vi "SP Simulate Filter Data.vi"() -> ()   [LabVIEW 2011]
uses:
  TypeDefs/SP Filter Type.ctl
panel:
  in  "Points":i32=181
  in  "Filter Type":T1=enum."Bandpass"
  out "X Values":i32[](array[numeric])=[0, 1, 2, 3, 4, 5, 6, 7, 8, 9, 10, 11, 12, 13, 14, 15, 16, 17, 18, 19, 20, 21, 22, 23, 24, 25, 26, 27, 28, 29, 30, 31, 32, 33, 34, 35, 36, 37, 38, 39, 40, 41, 42, 43, 44, 45, 46, 47, 48, 49, 50, 51, 52, 53, 54, 55, 56, 57, 58, 59, 60, 61, 62, 63, 64, 65, 66, 67, 68, 69, 70, 71, 72, 73, 74, 75, 76, 77, 78, 79, 80, 81, 82, 83, 84, 85, 86, 87, 88, 89, 90, 91, 92, 93, 94, 95, 96, 97, 98, 99, 100, 101, 102, 103, 104, 105, 106, 107, 108, 109, 110, 111, 112, 113, 114, 115, 116, 117, 118, 119, 120, 121, 122, 123, 124, 125, 126, 127, 128, 129, 130, 131, 132, 133, 134, 135, 136, 137, 138, 139, 140, 141, 142, 143, 144, 145, 146, 147, 148, 149, 150, 151, 152, 153, 154, 155, 156, 157, 158, 159, 160, 161, 162, 163, 164, 165, 166, 167, 168, 169, 170, 171, 172, 173, 174, 175, 176, 177, 178, 179, 180, 181, 182, 183, 184, 185, 186, 187, 188, 189, 190, 191, 192, 193, 194, 195, 196, 197, 198, 199, 200]
  out "Y Values":dbl[](array[numeric])=[-6.0, -6.0, -6.0, -6.0, -6.0, -6.0, -5.0, -4.0, -3.0, -2.0, -1.1855130217753456, -0.9392889870179464, -1.1861908270355541, -1.1367726789453658, -1.0393042985006378, -1.1729735369456953, -1.149385365911845, -1.1147598905277212, -0.8924252750804288, -0.852023103699543, -1.0009058190824704, -1.1663956046137898, -0.9001054770728154, -1.130526922084043, -1.1865443801186122, -0.8041911034172179, -1.1354203858940595, -0.9810522632655637, -0.8174498820167059, -0.8314370257909104, -1.1470623100787634, -0.8322674500080469, -1.139672707857633, -1.1197357445850977, -0.9958965192526265, -0.9621243610180682, -1.0476905954524998, -0.8242021422725134, -1.1913494829905178, -0.9868466615040767, -1.1724387156436977, -1.167152572929662, -0.8616430603149867, -1.140654519892024, -0.8539829798042038, -0.9647720176391821, -0.8587315795201268, -1.0567091604204648, -1.1192572463176262, -0.98486077165281, -1.0198831233507435, -1.0453093341117357, -0.9090367415909884, -0.9225201376325742, -0.8147168036204276, -1.107631457719548, -0.8164589952129693, -1.0035047526744438, -0.9758160980658377, -1.184168855175436, -0.842430499284283, -0.8295055444174504, -1.0907174559726884, -1.0463289127086592, -0.9523684118905202, -1.0086763511633476, -1.0058400904040357, -1.0432787022227192, -1.0004346015349277, -1.0142579998073553, -1.03249973907765, -1.1571657456698485, -0.8532729270453172, -0.830847736139528, -0.8321614396956182, -0.8398525997752223, -1.0931777911207057, -0.9353850412309945, -1.1033135631481505, -0.8359862020321329, -1.0100917820568274, -0.9437528106627642, -0.9234950263145335, -1.1828469590895319, -0.9732178966488259, -0.8312094485882828, -1.0994433199614881, -1.0711340736405945, -1.0161854731131412, -1.057480045668262, -1.0787569146834337, -1.150715751536042, -0.9306538142740585, -0.8619442330284444, -0.9498060661557108, -0.8760250798284357, -0.9560421828466075, -0.9006082904852345, -0.9198347197329708, -1.0706736281223097, -0.9910446023988131, -1.1659285288433643, -1.0742803411609738, -0.9771859793673917, -0.9576780670324955, -0.8573848364754029, -0.987301020537021, -0.815083398408206, -0.9954303077443712, -0.904598633827661, -0.917020167248773, -0.9859233342771836, -1.0886427454423657, -0.824049503823506, -0.9267990550448937, -1.0502624782226144, -0.9990423620181306, -0.9308037411565736, -1.1098504590826779, -1.159288905649198, -1.151169461672428, -0.8979842313793596, -1.0781960839410027, -1.0969866075108148, -1.113520232849719, -0.9242437596372882, -0.8322010245145881, -0.9131005811595208, -1.0502624924705835, -0.9860920827871864, -0.9686948150309891, -1.0436064687859832, -0.9811735822378999, -0.918340390858149, -1.087828104328058, -0.9581834504413268, -0.9790485893409894, -0.91805118027203, -0.8394459605871857, -1.0587904780939332, -1.1043679940556488, -1.103235946130976, -0.9329546049267435, -1.0870438319895284, -0.869725151175479, -0.8527906822295972, -0.8936094898921996, -0.8623252114256822, -1.0839364126457178, -1.1610235966131799, -1.0852518226294485, -0.8429280021959311, -1.1856901887322082, -1.052078336001964, -1.1295501456348471, -1.014702536100275, -1.107668899453921, -0.808453691868899, -1.0741488503523051, -1.0676276895458034, -0.8050463016216658, -0.9702859338685449, -1.037849817531343, -1.1042259704060462, -1.087009412780065, -0.9269022138105869, -0.8821968384650177, -0.9952550757996109, -1.0399315437270453, -1.1993212651287672, -1.1661312738652736, -1.0812208427752024, -1.1971807752359445, -1.1135450915006633, -0.8193764144655277, -0.9009947308628669, -0.8717741642808872, -1.007749740491375, -0.896481392578258, -0.964590014671117, -1.106404269705894, -1.0422703718848416, -0.9463098078312262, -1.0200691923673444, -1.056772196366392, -0.9059923317295363, -0.9680609411906224, -0.8086586664793829, -0.8983537306170685, -1.1283136612464237, -1.117694602097225, -2.0, -3.0, -4.0, -5.0, -6.0, -6.0, -6.0, -6.0, -6.0, -6.0]
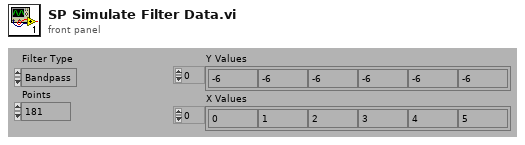
[diagram p1: front panel]
types:
  T1 = typedef "SP Filter Type.ctl" = enum16{"Lowpass", "Highpass", "Bandpass", "Bandstop"}
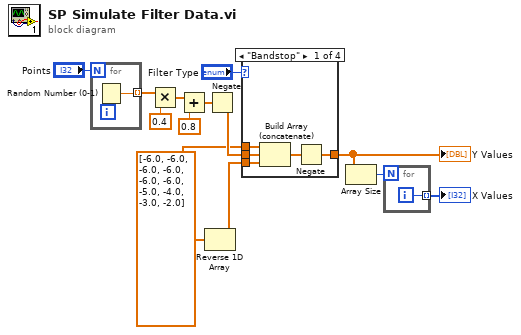
[diagram p0: block diagram]
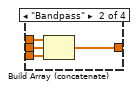
[diagram p2: hidden frame]
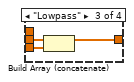
[diagram p3: hidden frame]
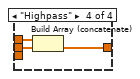
[diagram p4: hidden frame]
diagram:
  w4 = dbl[] [-6.0, -6.0, -6.0, -6.0, -6.0, -6.0, -5.0, -4.0, -3.0, -2.0] ("x+y")
  n1 = for {
    N: "Points" -> [_]
    tunnel: [w14] -> w12 mode=indexing
    n2 = Random Number (0-1)() -> (number: 0 to 1=w14:dbl)
  }
  n3 = Multiply(x=w12, y=0.4 ("number: 0 to 1")) -> (x*y=w10:dbl[])
  n4 = Add(x=w10, y=0.8 ("number: 0 to 1")) -> (x+y=w8:dbl[])
  n5 = Reverse 1D Array(array=w4) -> (reversed array=w3:dbl[])
  n6 = Negate(x=w8) -> (-x=w7:dbl[])
  n7 = case shown="\"Bandstop\"" "Filter Type" {
    tunnel: w7 -> [w19 w23 w26 w29]
    tunnel: w4 -> [w18 w22 _ w27]
    tunnel: w3 -> [w17 w21 w25 _]
    tunnel: [w15 w20 w24 w28] -> w2
    frame "Bandstop" {
      n8 = Build Array (concatenate)(w18, w19, w17) -> (w16:dbl[])
      n9 = Negate(x=w16) -> (-x=w15:dbl[])
    }
    frame "Bandpass" {
      n10 = Build Array (concatenate)(w22, w23, w21) -> (w20:dbl[])
    }
    frame "Lowpass" {
      n11 = Build Array (concatenate)(w26, w25) -> (w24:dbl[])
    }
    frame "Highpass" {
      n12 = Build Array (concatenate)(w27, w29) -> (w28:dbl[])
    }
  }
  "Y Values" <- w2
  n13 = Array Size(array=w2) -> (size(s)=w6:i32)
  n14 = for {
    N: w6 -> [_]
    tunnel: [w30] -> w5 mode=indexing
    i -> [w30]
  }
  "X Values" <- w5
